vi "projectShortener.vi"(6 "Site Specific String (Blank if Surrey)":string, 10 "fullProjectName":string) -> (2 "projectNameOut":string)   [LabVIEW 2022 SP3]
panel:
  # "Shortens project names which start with a number to just that number, if site is CPP\n\nIntended to deal with overly-long names which cause path length failures.\nNon-numeric first characters, or 9999 projects unaffected."
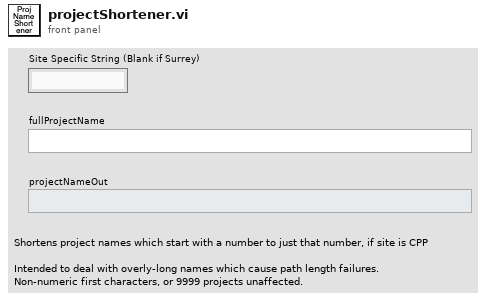
[diagram p1: front panel]
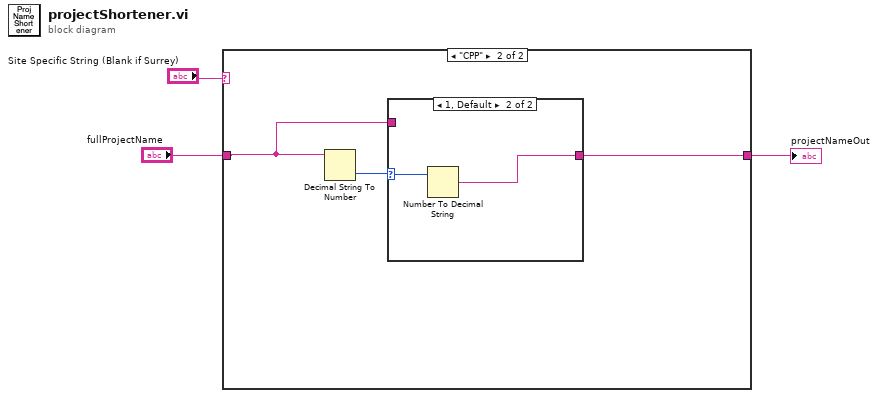
[diagram p0: block diagram]
diagram:
  n1 = case shown="\"CPP\"" "Site Specific String (Blank if Surrey)" {
    tunnel: "fullProjectName" -> [w4 w5]
    tunnel: [w4 w7] -> w1
    frame "False", Default {
    }
    frame "CPP" {
      n2 = Decimal String To Number(string=w5) -> (number=w6:i32)  [unwired: 2 in, 1 out]
      n3 = case shown="1, Default" w6 {
        selector: w6 -> [_ w9]
        tunnel: [w8 w10] -> w7
        tunnel: w5 -> [w8 _]
        frame 0, 9999 {
        }
        frame 1, Default {
          n4 = Number To Decimal String(number=w9) -> (decimal integer string=w10:string)  [unwired: 1 in]
        }
      }
    }
  }
  "projectNameOut" <- w1
